vi "port_code.vi"(8 "error in (no error)":errorcluster, 10 "Code to run":string, 11 "VISA Refnum in":refnum<visa-resource-name>) -> (0 "error out":errorcluster, 3 "VISA Refnum out":refnum<visa-resource-name>)   [LabVIEW 2024]
uses:
  <vilib>/Utility/error.llb/Trim Whitespace One-Sided.vi
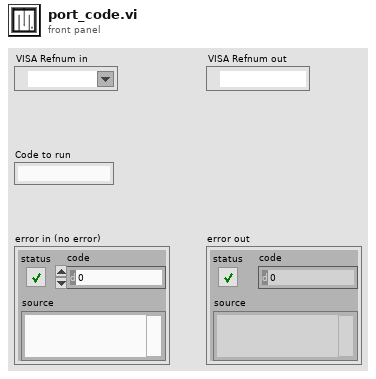
[diagram p1: front panel]
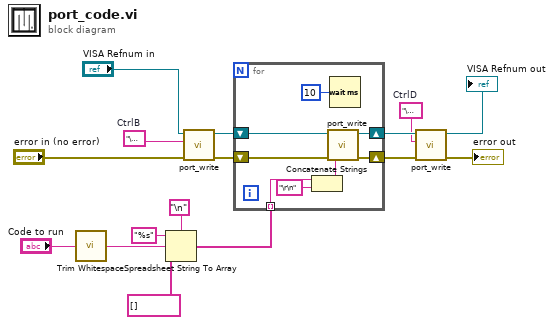
[diagram p0: block diagram]
diagram:
  w4 = "\u0005"  # CtrlB
  w3 = "\u0004"  # CtrlD
  n1 = call <vilib>:"Trim Whitespace.vi"("string"="Code to run") -> ("trimmed string"=w1:string)  [unwired: 1 in]
  n2 = Spreadsheet String To Array(delimiter (Tab)="\n" ("search string"), format string="%s", spreadsheet string=w1, array type (2D Dbl)=string[] []) -> (array=w2:string[])
  n3 = call <userlib>:"port_write.vi"("error in (no error)"="error in (no error)", "write buffer"=w4, "VISA Refnum in"="VISA Refnum in") -> ("error out"=w10:errorcluster, "VISA Refnum out"=w9:refnum<visa-resource-name>)  [unwired: 7 in]
  n4 = for {
    shift-right: [w22] -> w8
    shift-left: w10 -> [w24]
    shift-right: [w21] -> w7
    shift-left: w9 -> [w23]
    tunnel: w2 -> [w19] mode=indexing
    n5 = Concatenate Strings(w19, "\r\n" ("string")) -> (w18:string)
    n6 = call <userlib>:"port_write.vi"("error in (no error)"=w24, "write buffer"=w18, "VISA Refnum in"=w23) -> ("error out"=w22:errorcluster, "VISA Refnum out"=w21:refnum<visa-resource-name>)  [unwired: 7 in]
    n7 = Wait (ms)(milliseconds to wait=u32 10) -> ()  [unwired: 1 out]
  }
  n8 = call <userlib>:"port_write.vi"("error in (no error)"=w8, "write buffer"=w3, "VISA Refnum in"=w7) -> ("error out"=→"error out":errorcluster, "VISA Refnum out"=→"VISA Refnum out":refnum<visa-resource-name>)  [unwired: 7 in]
